vi "Stop Server.vi"(8 "error in":errorcluster, 11 "gRPC Server in":refnum<class "Servicer.lvclass">) -> (0 "error out":errorcluster)   [LabVIEW 2019, in "gRPC-servicer.lvlib" / "Servicer.lvclass"]
uses:
  Servicer.lvclass
  Servicer.lvclass/Servicer.ctl
  <vilib>/gRPC/LabVIEW gRPC Library/gprc-lvsupport-release.lvlib
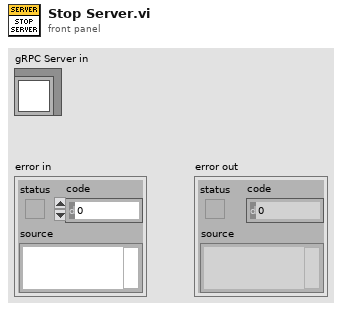
[diagram p1: front panel]
types:
  T1 = typedef "gprc-lvsupport-release.lvlib/grpcId.ctl" = u64
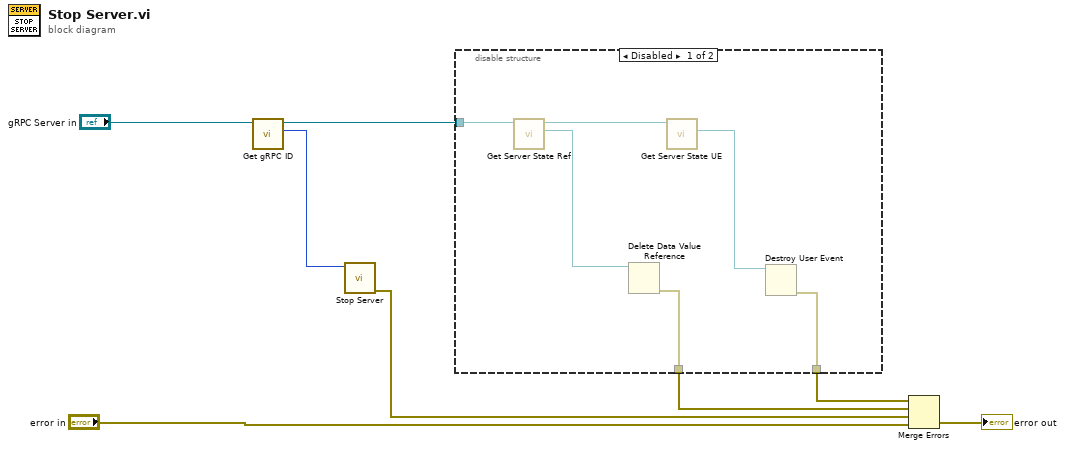
[diagram p0: block diagram]
diagram:
  n1 = call "Get gRPC ID.vi"("OOP Server in"="gRPC Server in") -> ("gRPC ID"=w2:T1, "OOP Server out"=w1:refnum<class "Servicer.lvclass">)  [unwired: 9 in]
  n2 = call <vilib>:"Stop Server.vi"("Server Id"=w2) -> ("error out"=w6:errorcluster)  [unwired: 10 in]
  n3 = disable-structure shown="Disabled" {
    disable-tunnel: w1 -> [w12 _]
    disable-tunnel: [w14 _] -> w5
    disable-tunnel: [w13 _] -> w4
    frame Disabled {
      n4 = call "Get Server State Ref.vi"("Template Server in"=w12) -> ("Server State Ref"=w10:refnum<data-value>, "Template Server out"=w11:refnum<class "Servicer.lvclass">)  [unwired: 9 in]
      n5 = Delete Data Value Reference(data value reference=w10) -> (error out=w14:errorcluster)  [unwired: 1 in, 1 out]
      n6 = call "Get Server State UE.vi"("Template Server in"=w11) -> ("Server Internal State UE"=w9:refnum<user-event>)  [unwired: 9 in, 1 out]
      n7 = Destroy User Event(user event=w9) -> (error out=w13:errorcluster)  [unwired: 1 in]
    }
    frame Enabled {
    }
  }
  n8 = Merge Errors(w4, w5, w6, "error in") -> (→"error out":errorcluster)
